vi "Check Ready.vi"(8 "error in (no error)":errorcluster, 9 "Timeout":i32, 11 "Enclave in":refnum<class "Enclave.lvclass">) -> (0 "error out":errorcluster, 1 "Remaining Timeout":i32, 3 "Enclave out":refnum<class "Enclave.lvclass">)   [LabVIEW 2022 SP3, in "Enclave.lvlib" / "Enclave.lvclass"]
uses:
  Enclave.lvclass
  Enclave.lvclass/Enclave.ctl
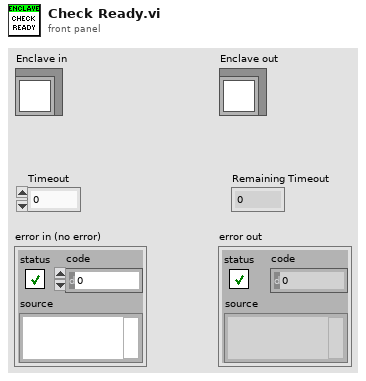
[diagram p1: front panel]
types:
  T1 = typedef "Enclave.lvlib/Writer Data.ctl" = cluster{"Queues":refnum<queue>[], "Lossy":bool, "Event":bool}
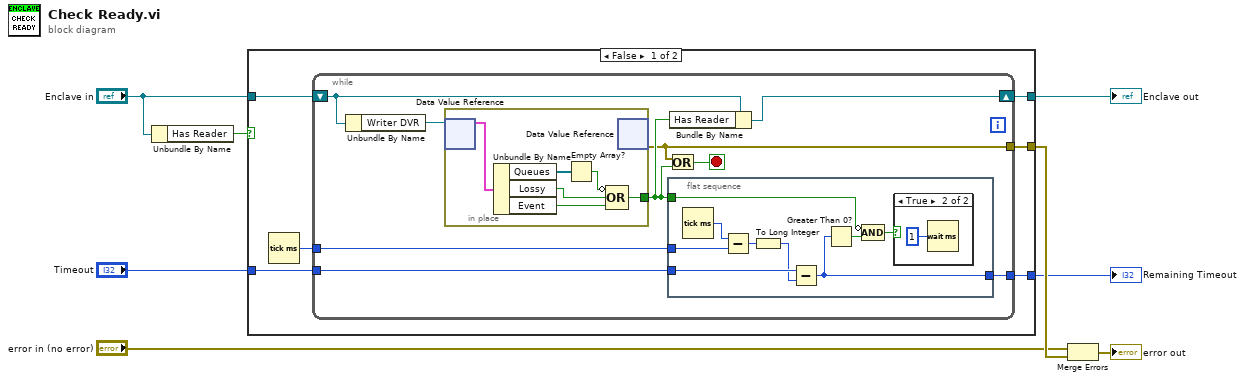
[diagram p0: block diagram]
diagram:
  n1 = Unbundle By Name("Enclave in") -> ("Has Reader"=w6:bool)
  n2 = case shown="False" w6 {
    tunnel: "Enclave in" -> [w14 w41]
    tunnel: [w12 w41] -> w4
    tunnel: "Timeout" -> [w13 w40]
    tunnel: [w10 w40] -> w2
    tunnel: [w9 _] -> w8
    frame False {
      n3 = Tick Count (ms)() -> (millisecond timer value=w11:u32)
      n4 = while {
        shift-right: [w23] -> w12
        shift-left: w14 -> [w22]
        tunnel: w13 -> [w19]
        tunnel: w11 -> [w20]
        tunnel: [w18] -> w10
        tunnel: [w15] -> w9
        stop <- w16 stop-if-true
        n5 = Unbundle By Name(w22) -> ("Writer DVR"=w21:refnum<data-value>)
        n6 = in-place {
          in-place-border: [w34] -> w17
          n7 = in-place-dvr #1(w21) -> (w39:T1)  [unwired: 1 out]
          n8 = Unbundle By Name(w39) -> ("Queues"=w36:refnum<queue>[], "Lossy"=w37:bool, "Event"=w38:bool)
          n9 = Empty Array?(array=w36) -> (empty?=w35:bool)
          n10 = Compound Arithmetic op=OR(invert w35, w37, w38) -> (w34:bool)
          n11 = in-place-dvr #1() -> (w15:errorcluster)  [unwired: 1 in, 1 out]
        }
        n12 = Or(x=w15, y=w17) -> (x .or. y?=w16:bool)
        n13 = flat-sequence {
          tunnel: w20 -> [w32]
          tunnel: w19 -> [w31]
          tunnel: [w30] -> w18
          tunnel: w17 -> [w24]
          frame #0 {
            n14 = Tick Count (ms)() -> (millisecond timer value=w29:u32)
            n15 = Subtract(x=w29, y=w32) -> (x-y=w28:u32)
            n16 = To Long Integer(number=w28) -> (32bit integer=w27:i32)
            n17 = Subtract(x=w31, y=w27) -> (x-y=w30:i32)
            n18 = Greater Than 0?(x=w30) -> (x > 0?=w26:bool)
            n19 = Compound Arithmetic op=AND(invert w24, w26) -> (w25:bool)
            n20 = case shown="True" w25 {
              frame False {
              }
              frame True {
                n21 = Wait (ms)(milliseconds to wait=u32 1) -> ()  [unwired: 1 out]
              }
            }
          }
        }
        n22 = Bundle By Name(cluster=w22, "Has Reader"=w17) -> (w23:refnum<class "Enclave.lvclass">)
      }
    }
    frame True {
    }
  }
  "Enclave out" <- w4
  "Remaining Timeout" <- w2
  n23 = Merge Errors("error in (no error)", w8) -> (→"error out":errorcluster)
